vi "Send Command.vi"(8 "error in":errorcluster, 9 "Value":variant, 10 "Command":string, 11 "Analog-Output in":refnum<class "Analog-Output.lvclass">) -> (0 "error out":errorcluster, 3 "Analog-Output out":refnum<class "Analog-Output.lvclass">)   [LabVIEW 2019, in "Analog-Output.lvlib" / "Analog-Output.lvclass"]
uses:
  Library/Analog-Output.lvclass
  C:/Users/Public/Documents/Development/builds/Engine/Engine.lvlibp/Project/Engine.lvclass
  C:/Users/Public/Documents/Development/builds/Engine/Monitored Actor.lvlibp/Monitored Actor/Monitored Actor/Monitored Actor.lvclass
  Analog-Output Messages/Set Voltage Msg/Set Voltage Msg.lvclass/Set Voltage Msg.ctl
  Analog-Output Messages/Write Active Channel Msg/Write Active Channel Msg.lvclass/Write Active Channel Msg.ctl
  Analog-Output Messages/Set Voltage by Name Msg/Set Voltage by Name Msg.lvclass/Set Voltage by Name Msg.ctl
  builds/Engine/Engine.lvlibp/Accessors/Read Self Q.vi
  builds/Engine/Monitored Actor.lvlibp/Monitored Actor/Monitored Actor/Read Actor Label.vi
  <vilib>/Utility/error.llb/Error Cluster From Error Code.vi
  builds/Engine/Actor Framework.lvlibp/1abvi3w/vi.lib/ActorFramework/Message Enqueuer/Enqueue.vi
  builds/Engine/Actor Framework.lvlibp/1abvi3w/vi.lib/ActorFramework/Message Enqueuer/Message Enqueuer.lvclass
  <vilib>/ErrorRing/Error Ring.xnode
  Analog-Output Messages/Set Voltage Msg/Set Voltage Msg.lvclass
  Analog-Output Messages/Write Active Channel Msg/Write Active Channel Msg.lvclass
  Analog-Output Messages/Set Voltage by Name Msg/Set Voltage by Name Msg.lvclass
  builds/Engine/Engine.lvlibp/Project/Engine.lvclass
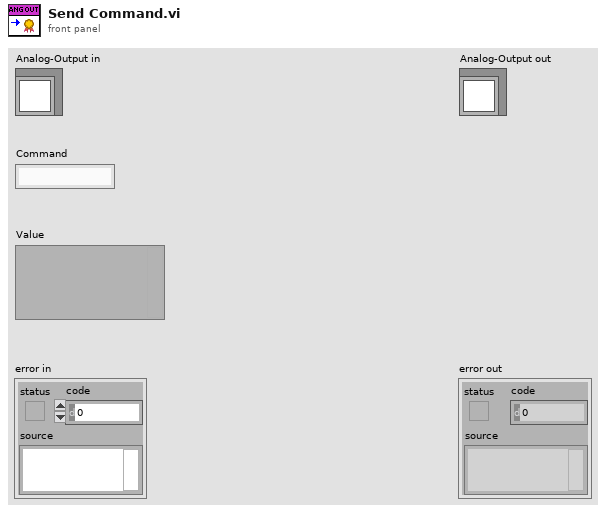
[diagram p1: front panel]
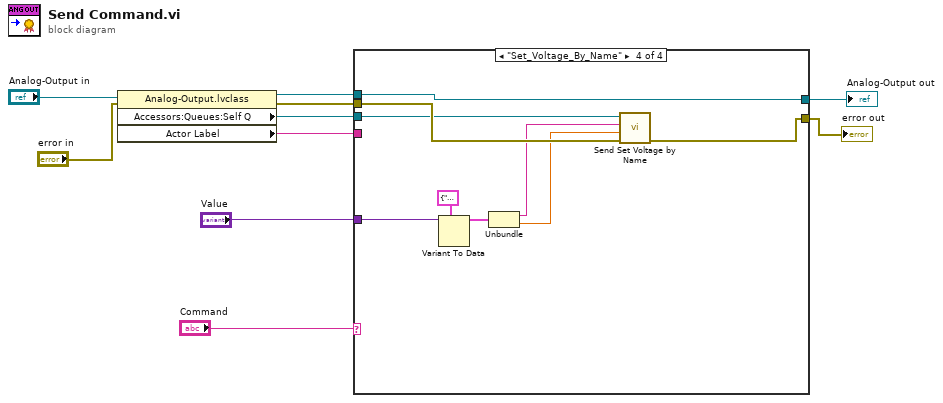
[diagram p0: block diagram]
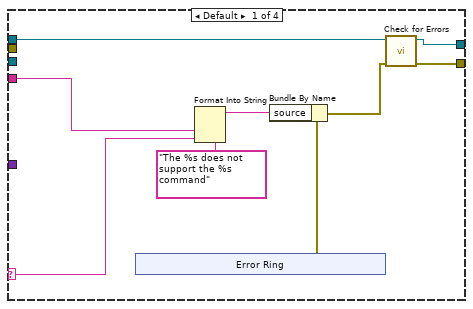
[diagram p2: hidden frame]
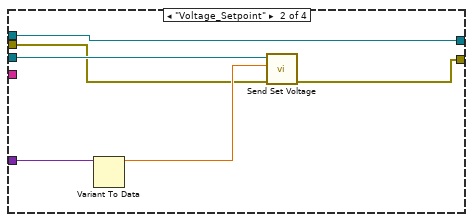
[diagram p3: hidden frame]
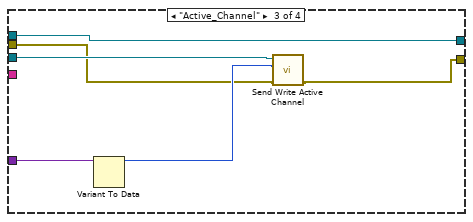
[diagram p4: hidden frame]
diagram:
  n1 = property class="Analog-Output.lvclass"(reference="Analog-Output in", error in="error in") -> (reference out=w4:refnum<class "Analog-Output.lvclass">, error out=w5:errorcluster, "Accessors:Queues:Self Q"=w1:refnum<class "Message Enqueuer.lvclass">, "Actor Label"=w7:string)
  n2 = case shown="\"Set_Voltage_By_Name\"" "Command" {
    selector: "Command" -> [w17 _ _ _]
    tunnel: "Value" -> [_ w29 w35 w44]
    tunnel: w7 -> [w18 _ _ _]
    tunnel: w5 -> [_ w24 w30 w42]
    tunnel: w4 -> [w15 w26 w34 w43]
    tunnel: [w12 w26 w34 w43] -> w3
    tunnel: [w11 w25 w33 w41] -> w2
    tunnel: w1 -> [_ w27 w32 w40]
    frame Default {
      n3 = xnode "Error Ring"() -> ("error out"=w13:errorcluster)
      n4 = Format Into String(format string="The %s does not support the %s command", w18, w17) -> (resulting string=w16:string)  [unwired: 2 in, 1 out]
      n5 = Bundle By Name(cluster=w13, "source"=w16) -> (w14:errorcluster)
      n6 = call "Check for Errors.vi"("error in"=w14, "Engine in"=w15) -> ("error out"=w11:errorcluster, "Engine out"=w12:refnum<class "Analog-Output.lvclass">)  [unwired: 8 in]
    }
    frame "Voltage_Setpoint" {
      n7 = Variant To Data(Variant=w29) -> (data=w28:dbl)  [unwired: 2 in, 1 out]
      n8 = call "Send Set Voltage.vi"("error in (no error)"=w24, "Voltage"=w28, "Message Enqueuer"=w27) -> ("error out"=w25:errorcluster)  [unwired: 7 in, 1 out]
    }
    frame "Active_Channel" {
      n9 = Variant To Data(Variant=w35) -> (data=w31:u32)  [unwired: 2 in, 1 out]
      n10 = call "Send Write Active Channel.vi"("error in (no error)"=w30, "Active Channel"=w31, "Message Enqueuer"=w32) -> ("error out"=w33:errorcluster)  [unwired: 7 in, 1 out]
    }
    frame "Set_Voltage_By_Name" {
      n11 = Variant To Data(type=cluster{"Name":string, "Voltage":dbl} {"Name"="", "Voltage"=0.0}, Variant=w44) -> (data=w38:cluster{"Name":string, "Voltage":dbl})  [unwired: 1 in, 1 out]
      n12 = Unbundle(w38) -> ("Name"=w37:string, "Voltage"=w36:dbl)
      n13 = call "Send Set Voltage by Name.vi"("error in (no error)"=w42, "Voltage"=w36, "Channel_Name"=w37, "Message Enqueuer"=w40) -> ("error out"=w41:errorcluster)  [unwired: 6 in, 1 out]
    }
  }
  "error out" <- w2
  "Analog-Output out" <- w3
